vi "Compressor.vi"(8 "error in (no error)":errorcluster, 10 "CompressorDevRef 2":T1={"DevStatus"={"status"=FALSE, "code"=0, "source"=""}, "DigitalInputDevRef"={"DevStatus"={"status"=FALSE, "code"=0, "source"=""}, "DIO Channel"=enum."Invalid", "Digital Module"=enum."Digital Module 1"}, "RelayDevRef"={"DevStatus"={"status"=FALSE, "code"=0, "source"=""}, "Relay Channel"=enum."Invalid", "Digital Module"=enum."Digital Module 1", "Relay Direction"=enum."Both directions"}}, 11 "CompressorDevRef":T1={"DevStatus"={"status"=FALSE, "code"=0, "source"=""}, "DigitalInputDevRef"={"DevStatus"={"status"=FALSE, "code"=0, "source"=""}, "DIO Channel"=enum."Invalid", "Digital Module"=enum."Digital Module 1"}, "RelayDevRef"={"DevStatus"={"status"=FALSE, "code"=0, "source"=""}, "Relay Channel"=enum."Invalid", "Digital Module"=enum."Digital Module 1", "Relay Direction"=enum."Both directions"}}) -> ()   [LabVIEW 2013]
doc: "Monitors the pressure switch and updates the relay of up to two compressors. Use the Start, Stop, and GetEnableState VIs to update the compressor state. Use this VI in parallel with the rest of the robot code. Do not place this VI in another loop or in the Teleop code.\n\nThis software is licensed. Open the labview\\readme\\WPI Robotics Library Open Source License.txt file for more information."
uses:
  <vilib>/Rock Robotics/WPI/Compressor/WPI_CompressorDevRef.ctl
  <vilib>/Rock Robotics/WPI/DigitalInput/WPI_DigitalInputDevRef.ctl
  <vilib>/Rock Robotics/SystemInterfaces/DIO/FPGA_DIOChannel.ctl
  <vilib>/Rock Robotics/SystemInterfaces/Typedef/FPGA_TypedefDigitalModule.ctl
  <vilib>/Rock Robotics/WPI/Relay/WPI_RelayDevRef.ctl
  <vilib>/Rock Robotics/SystemInterfaces/DIO/FPGA_DIORelayChannel.ctl
  <vilib>/Rock Robotics/WPI/Relay/WPI_RelayDirection.ctl
  <vilib>/Rock Robotics/WPI/Relay/WPI_RelayValue.ctl
panel:
  # "This VI loops and doesn't return.\nPlacing it into another loop will\nprevent that loop from iterating.\n\nPeriodic tasks is a good location for it."
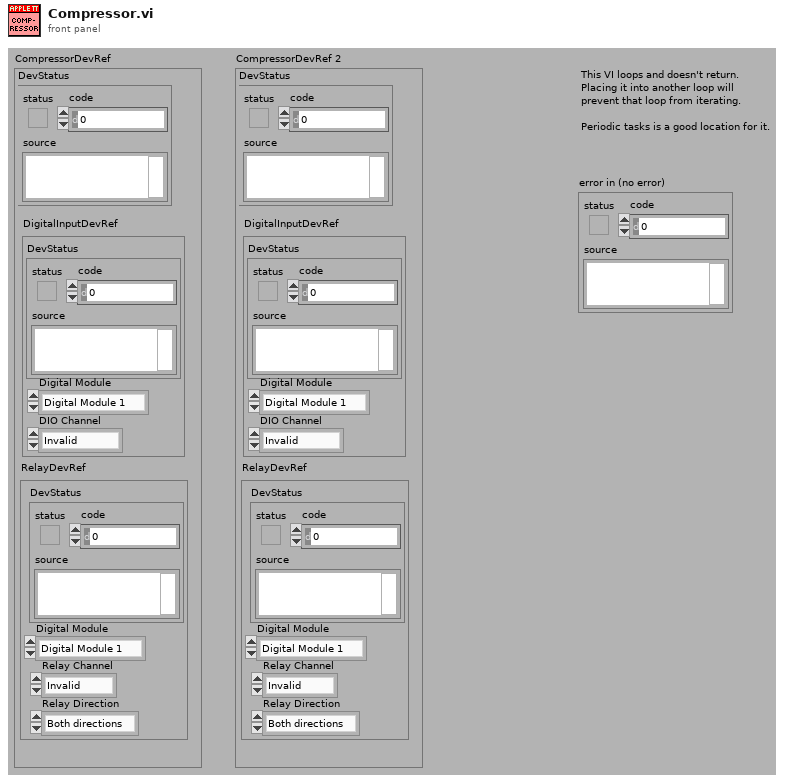
[diagram p1: front panel]
types:
  T1 = typedef "WPI_CompressorDevRef.ctl" = cluster{"DevStatus":errorcluster, "DigitalInputDevRef":T2, "RelayDevRef":T5}
  T2 = typedef "WPI_DigitalInputDevRef.ctl" = cluster{"DevStatus":errorcluster, "DIO Channel":T3, "Digital Module":T4}
  T3 = typedef "FPGA_DIOChannel.ctl" = enum8{"DIO 1", "DIO 2", "DIO 3", "DIO 4", "DIO 5", "DIO 6", "DIO 7", "DIO 8", "DIO 9", "DIO 10", "DIO 11", "DIO 12", "DIO 13", "DIO 14", "Invalid"}
  T4 = typedef "FPGA_TypedefDigitalModule.ctl" = enum16{"Digital Module 1", "Digital Module 2"}
  T5 = typedef "WPI_RelayDevRef.ctl" = cluster{"DevStatus":errorcluster, "Relay Channel":T6, "Digital Module":T4, "Relay Direction":T7}
  T6 = typedef "FPGA_DIORelayChannel.ctl" = enum8{"Relay 1", "Relay 2", "Relay 3", "Relay 4", "Relay 5", "Relay 6", "Relay 7", "Relay 8", "Invalid"}
  T7 = typedef "WPI_RelayDirection.ctl" = enum16{"Both directions", "Forward only", "Reverse only"}
  T8 = typedef "WPI_RelayValue.ctl" = enum16{"Off", "On", "Forward", "Reverse"}
  T9 = enum16{"Wait", "Clear", "Release", "Cock", "Reset"}
  T10 = typedef "WPI_MotorControlDeviceRef.ctl" = cluster{"DeviceStatus":errorcluster, "Type":enum16{"PWM", "CAN"}, "PWM":cluster{"Digital Module":T4, "PWM Channel":T11, "DeadBand":T12}, "CAN":cluster{"Device Number":u8, "Control Mode":T13, "Semaphore":T14, "Max Vout":dbl}, "Invert":bool, "TransformRef":T15, "InvTransformRef":T15}
  T11 = typedef "FPGA_DIOPWMChannel.ctl" = enum8{"PWM 1", "PWM 2", "PWM 3", "PWM 4", "PWM 5", "PWM 6", "PWM 7", "PWM 8", "PWM 9", "PWM 10", "Invalid"}
  T12 = typedef "WPI_PWMDeadband.ctl" = cluster{"Name":string, "maxPositivePwm":i32, "minPositivePwm":i32, "centerPwm":i32, "maxNegativePwm":i32, "minNegativePwm":i32, "angularRange":u16}
  T13 = typedef "WPI_CANJaguar_ControlMode.ctl" = enum8{"Percent VBus", "Current", "Speed", "Position", "Voltage"}
  T14 = typedef "Semaphore RefNum" = refnum<k1>
  T15 = typedef "WPI_PWMTransform_ConPane.ctl" = refnum<vi>
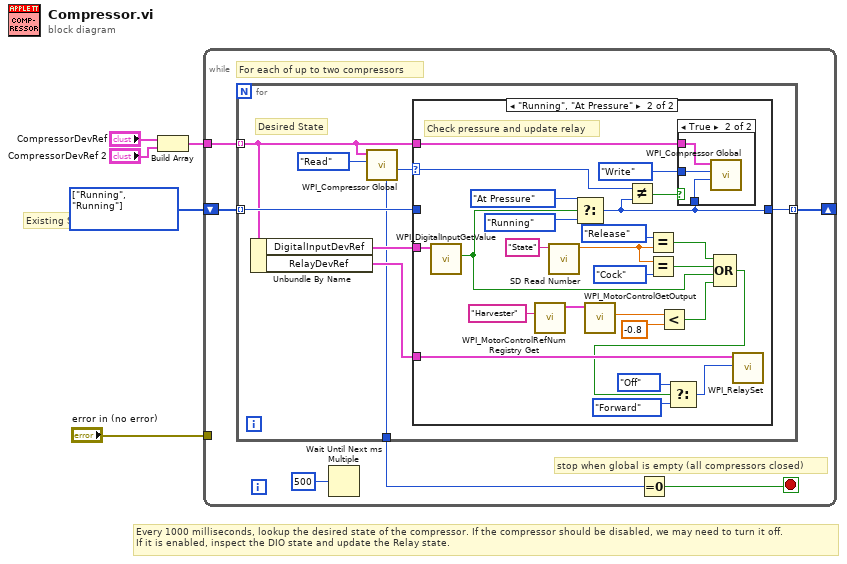
[diagram p0: block diagram]
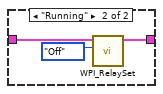
[diagram p3: hidden frame]
diagram:
  w1 = enum16{"Disabled", "Running", "At Pressure"}[] [enum."Running", enum."Running"] items=["Disabled", "Running", "At Pressure"]
  # "Every 1000 milliseconds, lookup the desired state of the compressor. If the compressor should be disabled, we may need to turn it off.\nIf it is enabled, inspect the DIO state and update the Relay state."
  # "Existing State"
  n1 = Build Array("CompressorDevRef", "CompressorDevRef 2") -> (w4:T1[])
  n2 = while {
    shift-right: [w9] -> _
    shift-left: w1 -> [w10]
    tunnel: "error in (no error)" -> [_]
    tunnel: w4 -> [w8]
    stop <- w6 stop-if-true
    # "stop when global is empty (all compressors closed)"
    # "For each of up to two compressors"
    n3 = for {
      tunnel: w10 -> [w19] mode=indexing
      tunnel: [w18] -> w9 mode=indexing
      tunnel: w8 -> [w13] mode=indexing
      tunnel: [w12] -> w7
      # "Desired State"
      n4 = Unbundle By Name(w13) -> ("DigitalInputDevRef"=w15:T2, "RelayDevRef"=w14:T5)
      n5 = call <vilib>:"WPI_Compressor Global.vi"("Operation"=enum16{"Read", "Write", "Add", "Remove"}."Read", "CompressorDevRef"=w13) -> ("Compressor State Out"=w16:enum16{"Disabled", "Running", "At Pressure"}, "Compressor Count"=w12:u8)  [unwired: 8 in]
      n6 = case shown="\"Running\", \"At Pressure\"" w16 {
        selector: w16 -> [w20 w40]
        tunnel: w15 -> [_ w51]
        tunnel: w14 -> [w22 w50]
        tunnel: w19 -> [w21 _]
        tunnel: [w20 w41] -> w18
        tunnel: w13 -> [_ w43]
        frame "Disabled", Default {
          n7 = case shown="Default" w21 {
            tunnel: w22 -> [w23 w25]
            tunnel: [w23 w24] -> _
            frame Default {
            }
            frame "Running" {
              n8 = call <vilib>:"WPI_RelaySet.vi"("RelayValue"=WPI_RelayValue."Off", "RelayDevRef"=w25) -> ("RelayDevRef"=w24:T5)  [unwired: 1 in, 8 out]
            }
          }
        }
        frame "Running", "At Pressure" {
          # "Check pressure and update relay"
          n9 = call <vilib>:"WPI_DigitalInputGetValue.vi"("DigitalInputDevRef"=w51) -> ("Value"=w29:bool)  [unwired: 1 in, 9 out]
          n10 = call <vilib>:"WPI_MotorControlRefNum Registry Get.vi"("refnum name"="Harvester") -> ("MotorControlDevRef"=w36:T10)  [unwired: 9 in, 1 out]
          n11 = call <vilib>:"SD Read Number.vi"("Name"="State") -> ("Numeric"=w33:dbl)  [unwired: 8 in, 2 out]
          n12 = Select(t=enum16{"Disabled", "Running", "At Pressure"}."At Pressure" ("Compressor State"), s=w29, f=enum16{"Disabled", "Running", "At Pressure"}."Running" ("Compressor State")) -> (s? t:f=w41:enum16{"Disabled", "Running", "At Pressure"})
          n13 = call <vilib>:"WPI_MotorControlGetOutput.vi"("MotorControlDevRef"=w36) -> ("Output"=w38:dbl)  [unwired: 8 in, 2 out]
          n14 = Not Equal?(x=w40, y=w41) -> (x != y?=w42:bool)
          n15 = Equal?(x=T9."Release", y=w33) -> (x = y?=w31:bool)
          n16 = Equal?(x=w33, y=T9."Cock" ("x")) -> (x = y?=w30:bool)
          n17 = Less?(x=w38, y=-0.8) -> (x < y?=w28:bool)
          n18 = case shown="True" w42 {
            tunnel: w41 -> [_ w54]
            tunnel: enum16{"Read", "Write", "Add", "Remove"}."Write" ("Operation") -> [_ w53]
            tunnel: w43 -> [_ w52]
            frame False {
            }
            frame True {
              n19 = call <vilib>:"WPI_Compressor Global.vi"("Compressor State In"=w54, "Operation"=w53, "CompressorDevRef"=w52) -> ()  [unwired: 7 in, 2 out]
            }
          }
          n20 = Compound Arithmetic op=OR(w31, w30, w29, w28) -> (w27:bool)
          n21 = Select(t=WPI_RelayValue."Off" ("RelayValue"), s=w27, f=WPI_RelayValue."Forward" ("RelayValue")) -> (s? t:f=w47:T8)
          n22 = call <vilib>:"WPI_RelaySet.vi"("RelayValue"=w47, "RelayDevRef"=w50) -> ()  [unwired: 1 in, 9 out]
        }
      }
    }
    n23 = Wait Until Next ms Multiple(millisecond multiple=u32 500 ("timeout in ms (0)")) -> ()  [unwired: 1 out]
    n24 = Equal To 0?(x=w7) -> (x = 0?=w6:bool)
  }
